vi "Lock Front Panel.vi"(8 "error in":errorcluster, 10 "Lock?":bool, 11 "4124 in":refnum<class "4124.lvclass">) -> (0 "error out":errorcluster, 3 "4124 out":refnum<class "4124.lvclass">)   [LabVIEW 2018, in "4124.lvlib" / "4124.lvclass"]
doc: "This VI allows the program to lock out front panel controls or unlock them."
uses:
  4124.lvclass
  <instrlib>/NI RMX-412x Power Supplies/NI RMX-412x Power Supplies.lvlib
  builds/Power_Supply.lvlibp/Power Supply.lvclass
  C:/Users/Ron.Dexter.LUMINARTECH/Desktop/builds/Power_Supply.lvlibp/Power Supply.lvclass
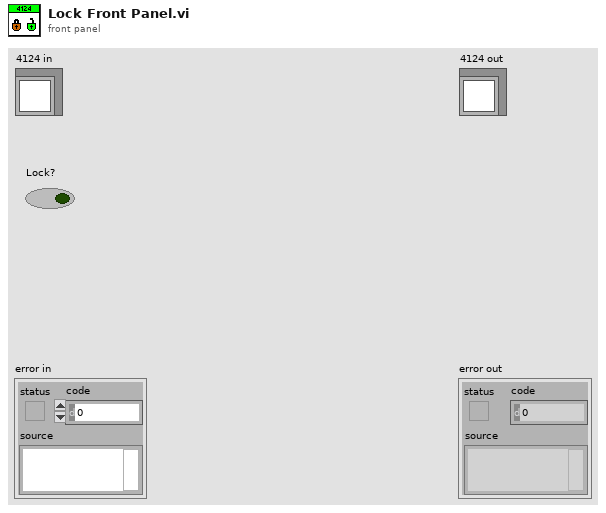
[diagram p1: front panel]
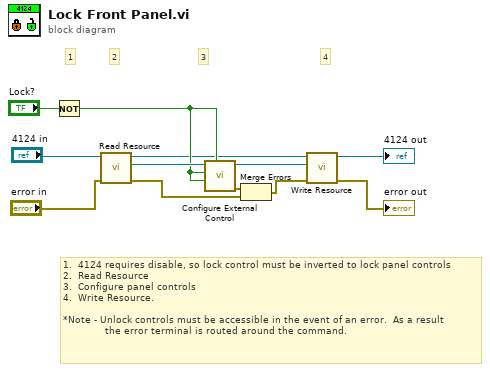
[diagram p0: block diagram]
diagram:
  # "1.  4124 requires disable, so lock control must be inverted to lock panel controls\n2.  Read Resource\n3.  Configure panel controls\n4.  Write Resource.\n\n*Note - Unlock controls must be accessible in the event of an error.  As a result\n              the error terminal is routed around the command."
  # "4"
  # "3"
  # "2"
  # "1"
  n1 = Not(x="Lock?") -> (.not. x?=w9:bool)
  n2 = call "Read Resource.vi"("error in"="error in", "Power Supply in"="4124 in") -> ("error out"=w1:errorcluster, "Resource"=w11:refnum<visa-resource-name>, "Power Supply out"=w8:refnum<class "4124.lvclass">)  [unwired: 7 in]
  n3 = call <instrlib>:"Configure External Control.vi"("Enable External Output Control (F: Disable)"=w9, "Enable External Voltage Control (F: Disable)"=w9, "Enable External Current Control (F: Disable)"=w9, "VISA resource name"=w11) -> ("error out"=w4:errorcluster, "VISA resource name out"=w7:refnum<visa-resource-name>)  [unwired: 6 in]
  n4 = Merge Errors(w4, w1) -> (w2:errorcluster)
  n5 = call "Write Resource.vi"("error in"=w2, "Resource"=w7, "Power Supply in"=w8) -> ("error out"=→"error out":errorcluster, "Power Supply out"=→"4124 out":refnum<class "4124.lvclass">)  [unwired: 7 in]
